vi "Create Process Events.vi"(8 "error in (no error)":errorcluster, 11 "Bar in":refnum<class "Bar.lvclass">) -> (0 "error out":errorcluster, 3 "Bar out":refnum<class "Bar.lvclass">)   [LabVIEW 2015, in "Simple Progress Bar.lvlib" / "Bar.lvclass"]
uses:
  Bar.lvclass
  Process Events.ctl
  Bar.lvclass/Bar.ctl
  Simple Progress Bar.lvlib
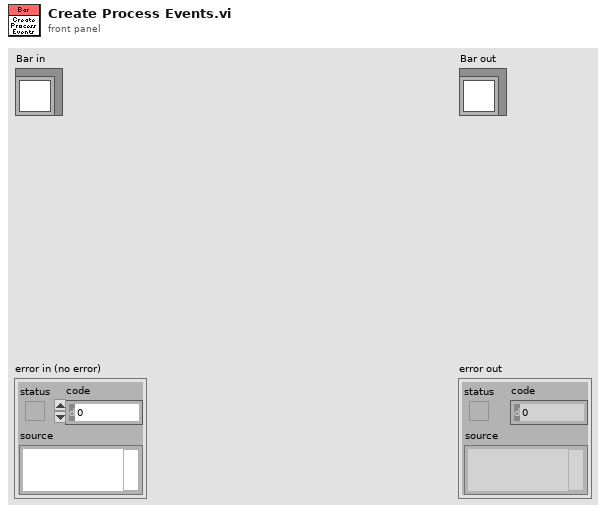
[diagram p1: front panel]
types:
  T1 = typedef "Simple Progress Bar.lvlib/Process Events.ctl" = cluster{"Explorer":refnum<user-event>, "Finished":refnum<user-event>, "Aborted":refnum<user-event>, "New Job":refnum<user-event>, "Item Status":refnum<user-event>, "Item Progression":refnum<user-event>, "Error":refnum<user-event>}
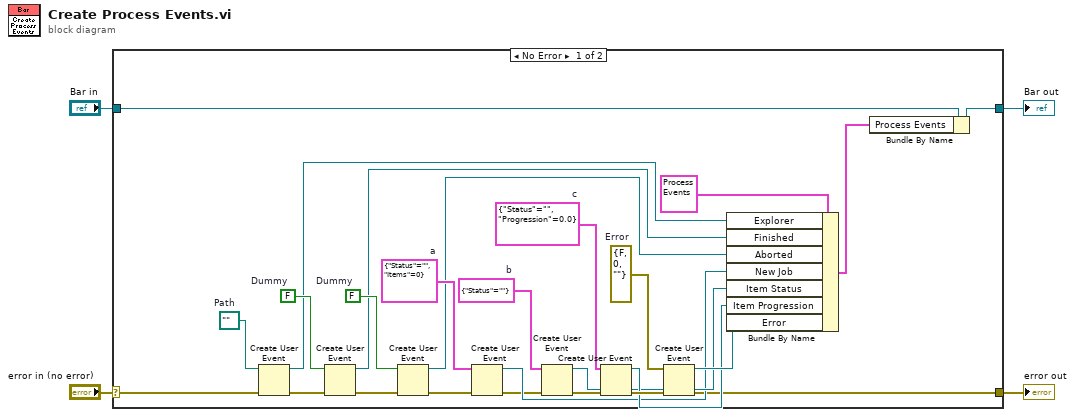
[diagram p0: block diagram]
diagram:
  n1 = case shown="No Error" "error in (no error)" {
    selector: "error in (no error)" -> [w8 w32]
    tunnel: [w7 w32] -> w3
    tunnel: [w6 w31] -> w1
    tunnel: "Bar in" -> [w30 w31]
    frame No Error {
      w28 = errorcluster {"status"=FALSE, "code"=0, "source"=""}  # Error
      w21 = cluster{"Status":string, "Items":i32} {"Status"="", "Items"=0}  # a
      w22 = cluster{"Status":string} {"Status"=""}  # b
      w17 = path ""  # Path
      w15 = FALSE  # Dummy
      w14 = FALSE  # Dummy
      w23 = cluster{"Status":string, "Progression":dbl} {"Status"="", "Progression"=0.0}  # c
      n2 = Create User Event(user event datatype=w17, error in=w8) -> (user event=w9:refnum<user-event>, error out=w10:errorcluster)
      n3 = Create User Event(user event datatype=w14, error in=w10) -> (user event=w12:refnum<user-event>, error out=w11:errorcluster)
      n4 = Create User Event(user event datatype=w15, error in=w11) -> (user event=w13:refnum<user-event>, error out=w18:errorcluster)
      n5 = Create User Event(user event datatype=w21, error in=w18) -> (user event=w24:refnum<user-event>, error out=w19:errorcluster)
      n6 = Create User Event(user event datatype=w22, error in=w19) -> (user event=w25:refnum<user-event>, error out=w20:errorcluster)
      n7 = Create User Event(user event datatype=w23, error in=w20) -> (user event=w26:refnum<user-event>, error out=w27:errorcluster)
      n8 = Create User Event(user event datatype=w28, error in=w27) -> (user event=w29:refnum<user-event>, error out=w7:errorcluster)
      n9 = Bundle By Name(cluster=T1 {"Explorer"=refnum, "Finished"=refnum, "Aborted"=refnum, "New Job"=refnum, "Item Status"=refnum, "Item Progression"=refnum, "Error"=refnum} ("Process Events"), "Explorer"=w9, "Finished"=w12, "Aborted"=w13, "New Job"=w24, "Item Status"=w25, "Item Progression"=w26, "Error"=w29) -> (w5:T1)
      n10 = Bundle By Name(cluster=w30, "Process Events"=w5) -> (w6:refnum<class "Bar.lvclass">)
    }
    frame Error {
    }
  }
  "error out" <- w3
  "Bar out" <- w1
